vi "chassis-speed-test.vi"(8 "error in (no error)":errorcluster) -> (0 "error out":errorcluster, 3 "Test Passed":bool)   [LabVIEW 2019]
uses:
  <vilib>/Rock Robotics/WPI/ThirdParty/JAS_Junk/TrajLib/Conv_Deg_Radians.vi
  <vilib>/Rock Robotics/WPI/ThirdParty/JAS_Junk/TrajLib/Rotation2d_CreateAngle.vi
  <vilib>/Rock Robotics/WPI/ThirdParty/JAS_Junk/TrajLib/Rotation2d_GetCos.vi
  <vilib>/Rock Robotics/WPI/ThirdParty/JAS_Junk/TrajLib/Rotation2d_GetSin.vi
  <vilib>/Rock Robotics/WPI/ThirdParty/JAS_Junk/TrajLib/ChassisSpeeds_New.vi
  <vilib>/Rock Robotics/WPI/ThirdParty/JAS_Junk/TrajLib/Trajectory_Library.lvlib
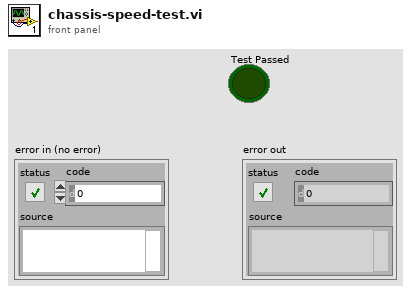
[diagram p1: front panel]
types:
  T1 = typedef "Trajectory_Library.lvlib/ROTATION2D.ctl" = cluster{"VALUE":dbl, "COS":dbl, "SIN":dbl}
  T2 = typedef "Trajectory_Library.lvlib/CHASSIS_SPEEDS.ctl" = cluster{"vX":dbl, "vY":dbl, "vOmega":dbl}
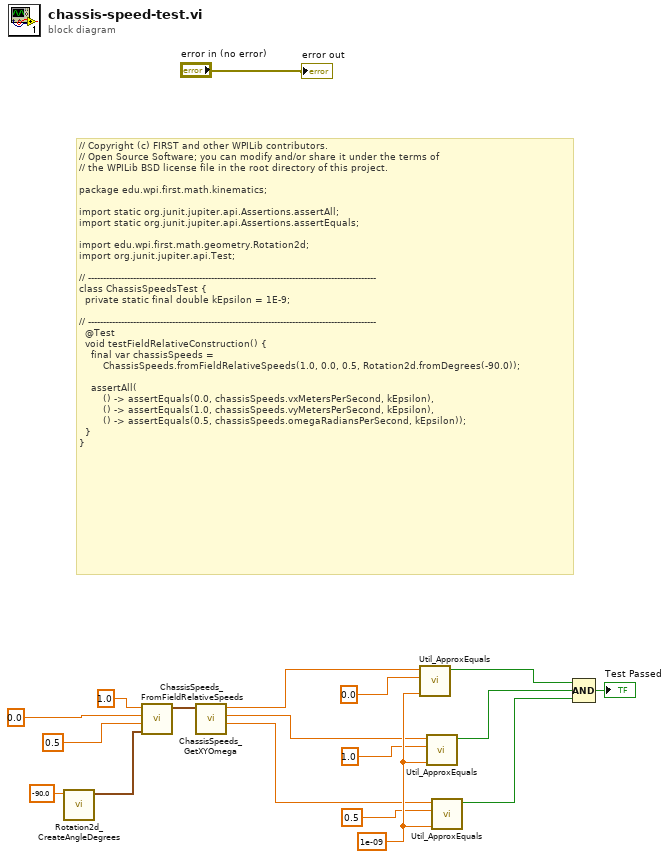
[diagram p0: block diagram]
diagram:
  w13 = 1e-09 ("Tolerance")
  # "// Copyright (c) FIRST and other WPILib contributors.\n// Open Source Software; you can modify and/or share it under the terms of\n// the WPILib BSD license file in the root directory of this project.\n\npackage edu.wpi.first.math.kinematics;\n\nimport static org.junit.jupiter.api.Assertions.assertAll;\nimport static org.junit.jupiter.api.Assertions.assertEquals;\n\nimport edu.wpi.first.math.geometry.Rotation2d;\nimport org.junit.jupiter.api.Test;\n\n// ------------------------------------------------------------------------------------------------\nclass ChassisSpeedsTest {\n  private static final double kEpsilon = 1E-9;\n\n// ------------------------------------------------------------------------------------------------\n  @Test\n  void testFieldRelativeConstruction() {\n    final var chassisSpeeds =\n        ChassisSpeeds.fromFieldRelativeSpeeds(1.0, 0.0, 0.5, Rotation2d.fromDegrees(-90.0));\n\n    assertAll(\n        () -> assertEquals(0.0, chassisSpeeds.vxMetersPerSecond, kEpsilon),\n        () -> assertEquals(1.0, chassisSpeeds.vyMetersPerSecond, kEpsilon),\n        () -> assertEquals(0.5, chassisSpeeds.omegaRadiansPerSecond, kEpsilon));\n  }\n}"
  n1 = call <vilib>:"Rotation2d_CreateAngleDegrees.vi"("Angle_Degrees"=-90.0) -> ("ROTATION"=w16:T1)  [unwired: 10 in]
  n2 = call <vilib>:"ChassisSpeeds_FromFieldRelativeSpeeds.vi"("RobotAngle"=w16, "Omega"=0.5, "vY"=0.0, "vX"=1.0) -> ("CHASSIS"=w5:T2)  [unwired: 7 in]
  n3 = call <vilib>:"ChassisSpeeds_GetXYOmega.vi"("CHASSIS"=w5) -> ("vAngular"=w2:dbl, "vY"=w3:dbl, "vX"=w4:dbl)  [unwired: 8 in]
  n4 = call <vilib>:"Util_ApproxEquals.vi"("Tolerance"=w13, "Value 2"=0.0, "Value 1"=w4) -> ("ApproxEquals"=w9:bool)  [unwired: 8 in]
  n5 = call <vilib>:"Util_ApproxEquals.vi"("Tolerance"=w13, "Value 2"=1.0, "Value 1"=w3) -> ("ApproxEquals"=w8:bool)  [unwired: 8 in]
  n6 = call <vilib>:"Util_ApproxEquals.vi"("Tolerance"=w13, "Value 2"=0.5, "Value 1"=w2) -> ("ApproxEquals"=w7:bool)  [unwired: 8 in]
  n7 = Compound Arithmetic op=AND(w9, w8, w7) -> (→"Test Passed":bool)
  "error out" <- "error in (no error)"
